vi "Test Valid Write.vi"() -> ()   [LabVIEW 2024]
uses:
  Mock Sift Proxy Server/Mock Sift Proxy Server.lvclass
  Sift API/Sift Client.lvclass
  Sift API/Types/Data Type.ctl
  Sift Client.lvlib
panel:
  out "Server Error":errorcluster
  out "Success 2":bool
  out "Error 2":errorcluster
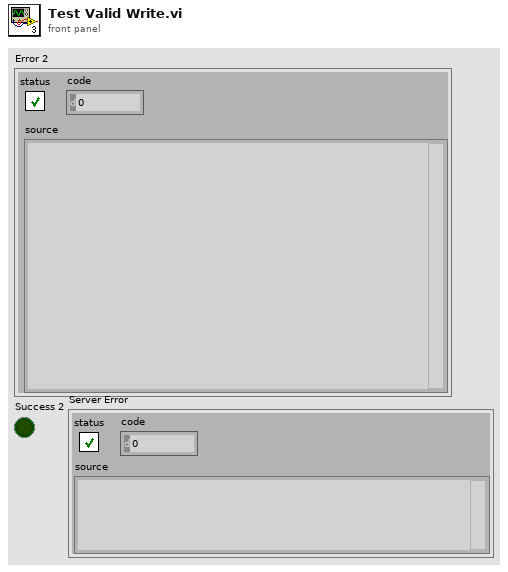
[diagram p1: front panel]
types:
  T1 = typedef "Sift Client.lvlib/Data Type.ctl" = enum8{"double", "float", "uint64", "int64", "uint32", "int32", "bool", "bit field", "enum"}
  T2 = typedef "Sift Client.lvlib/Timestamp.ctl" = cluster{"seconds":i64, "nanos":i32}
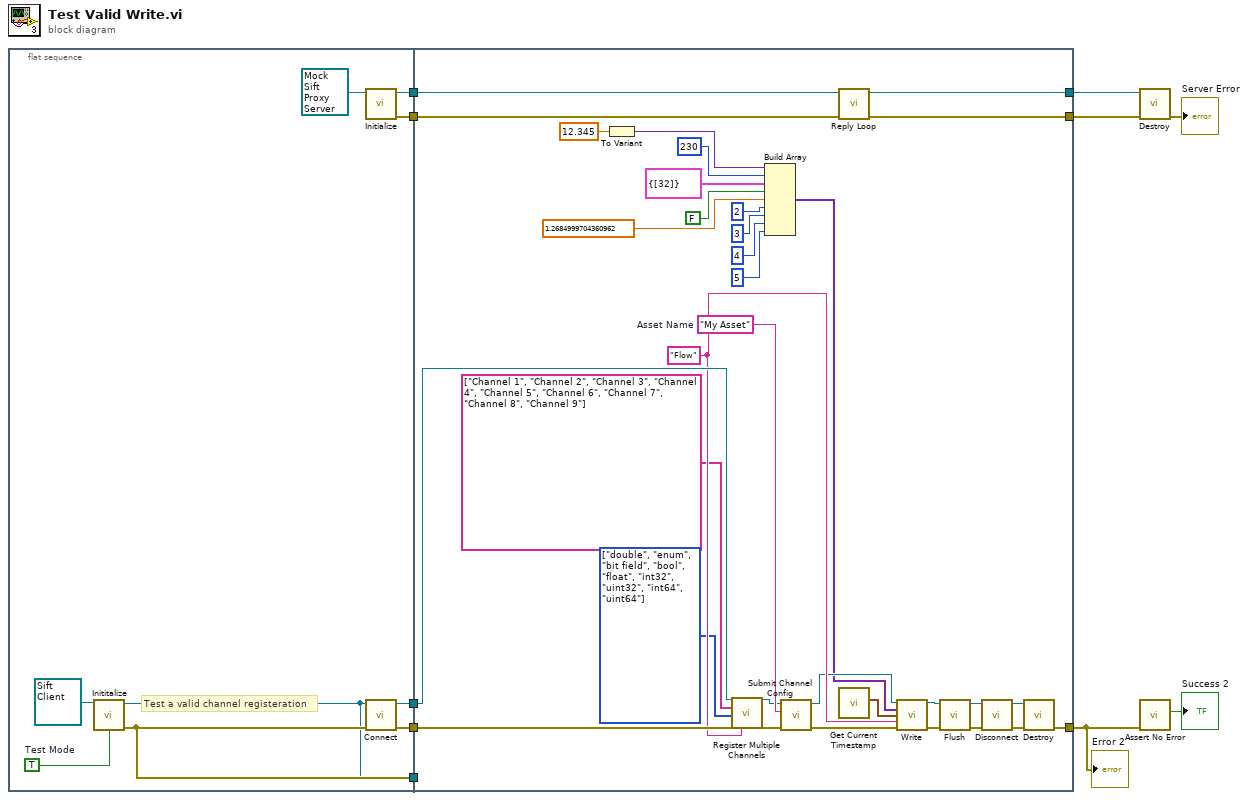
[diagram p0: block diagram]
diagram:
  n1 = flat-sequence {
    tunnel: [w19] -> w11
    tunnel: [w16] -> w10
    tunnel: [w15] -> w9
    tunnel: [w14] -> w8
    tunnel: [w13] -> w7
    tunnel: [w12] -> w6
    tunnel: [w48] -> w5
    tunnel: w11 -> [w49]
    tunnel: [w52] -> w1
    tunnel: w10 -> [_]
    tunnel: w9 -> [_]
    tunnel: w8 -> [w47]
    tunnel: w7 -> [w46]
    tunnel: w6 -> [w43]
    tunnel: [w42] -> w4
    frame #0 {
      w17 = TRUE  # Test Mode
      # "Test a valid channel registeration"
      n2 = call-dynamic "Inititalize.vi"("Sift Client in"=refnum<class "Sift Client.lvclass"> refnum ("Sift Client.lvlib:Sift Client.lvclass"), "Test Mode"=w17) -> ("Sift Client out"=w15:refnum<class "Sift Client.lvclass">, "error out"=w16:errorcluster)  [unwired: 12 in]
      n3 = call-dynamic "Initialize.vi"("Mock Sift Proxy Server in"=refnum<class "Mock Sift Proxy Server.lvclass"> refnum ("Mock Sift Proxy Server.lvclass")) -> ("error out"=w12:errorcluster, "Mock Sift Proxy Server out"=w19:refnum<class "Mock Sift Proxy Server.lvclass">)  [unwired: 9 in]
      n4 = call-dynamic "Connect.vi"("error in (no error)"=w16, "Sift Client in"=w15) -> ("error out"=w14:errorcluster, "Sift Client out"=w13:refnum<class "Sift Client.lvclass">)  [unwired: 7 in, 1 out]
    }
    frame #1 {
      w36 = T1[] [enum."double", enum."enum", enum."bit field", enum."bool", enum."float", enum."int32", enum."uint32", enum."int64", enum."uint64"] items=["double", "float", "uint64", "int64", "uint32", "int32", "bool", "bit field", "enum"]
      w51 = "My Asset"  # Asset Name
      w40 = "Flow" ("Flow Name")
      n5 = To Variant(anything=12.345) -> (Variant=w35:variant)
      n6 = call "Register Multiple Channels.vi"("Sift Client in"=w46, "Names"=string[] ["Channel 1", "Channel 2", "Channel 3", "Channel 4", "Channel 5", "Channel 6", "Channel 7", "Channel 8", "Channel 9"], "Data Types"=w36, "error in (no error)"=w47, "Flow Name"=w40) -> ("Sift Client out"=w50:refnum<class "Sift Client.lvclass">, "error out"=w53:errorcluster)  [unwired: 21 in]
      n7 = Build Array(w35, 230, cluster{u8[]} {[32]}, FALSE, sgl 1.2685, 2, 3, 4, 5) -> (w25:variant[])
      n8 = call-dynamic "Submit Channel Config.vi"("error in (no error)"=w53, "Asset Name"=w51, "Sift Client in"=w50) -> ("error out"=w38:errorcluster, "Sift Client out"=w39:refnum<class "Sift Client.lvclass">)  [unwired: 7 in]
      n9 = call-dynamic "Reply Loop.vi"("error in (no error)"=w43, "Mock Sift Proxy Server in"=w49) -> ("error out"=w42:errorcluster, "Mock Sift Proxy Server out"=w48:refnum<class "Mock Sift Proxy Server.lvclass">)  [unwired: 8 in]
      n10 = call "Get Current Timestamp.vi"() -> ("Timestamp"=w41:T2)  [unwired: 11 in]
      n11 = call-dynamic "Write.vi"("Sift Client in"=w39, "Values"=w25, "Timestamp"=w41, "Flow Name"=w40, "error in (no error)"=w38) -> ("Sift Client out"=w24:refnum<class "Sift Client.lvclass">, "error out"=w22:errorcluster)  [unwired: 9 in]
      n12 = call-dynamic "Flush.vi"("error in (no error)"=w22, "Sift Client in"=w24) -> ("error out"=w21:errorcluster, "Sift Client out"=w23:refnum<class "Sift Client.lvclass">)  [unwired: 7 in, 1 out]
      n13 = call-dynamic "Disconnect.vi"("error in (no error)"=w21, "Sift Client in"=w23) -> ("error out"=w44:errorcluster, "Sift Client out"=w45:refnum<class "Sift Client.lvclass">)  [unwired: 8 in]
      n14 = call-dynamic "Destroy.vi"("error in (no error)"=w44, "Sift Client in"=w45) -> ("error out"=w52:errorcluster)  [unwired: 8 in, 1 out]
    }
  }
  n15 = call-dynamic "Destroy.vi"("error in (no error)"=w4, "Mock Sift Proxy Server in"=w5) -> ("error out"=→"Server Error":errorcluster)  [unwired: 8 in, 1 out]
  n16 = call "Assert No Error.vi"("Error"=w1) -> ("Success"=→"Success 2":bool)  [unwired: 10 in]
  "Error 2" <- w1
